vi "Get transfer function.vi"() -> (0 "Continue? (T=yes)":bool=TRUE, 1 "Function for all neurons":enum16{"Linear", "Sigmoid", "Tangent hyp."}(ring)=enum."Sigmoid")   [LabVIEW 2010]
panel:
  in  "Function for all neurons":enum16{"Linear", "Sigmoid", "Tangent hyp."}(ring)=enum."Sigmoid"
  in  "Exit":bool
  in  "OK":bool
  # "Select transfer function..."
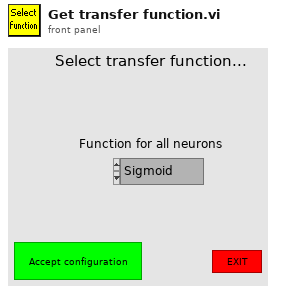
[diagram p1: front panel]
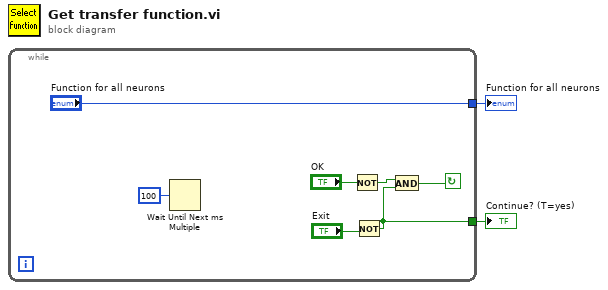
[diagram p0: block diagram]
diagram:
  n1 = while {
    tunnel: ["Function for all neurons"] -> w1
    tunnel: [w5] -> w2
    stop <- w6 continue-if-true
    n2 = Wait Until Next ms Multiple(millisecond multiple=u32 100) -> ()  [unwired: 1 out]
    n3 = Not(x="OK") -> (.not. x?=w8:bool)
    n4 = Not(x="Exit") -> (.not. x?=w5:bool)
    n5 = And(x=w8, y=w5) -> (x .and. y?=w6:bool)
  }
  "Continue? (T=yes)" <- w2
  "Function for all neurons" <- w1
